vi "Read Mode.vi"(8 "error in (no error)":errorcluster, 11 "Multimeter in":refnum<class "Multimeter.lvclass">) -> (0 "error out":errorcluster, 2 "Mode":T1, 3 "Multimeter out":refnum<class "Multimeter.lvclass">)   [LabVIEW 2019, in "Multimeter.lvlib" / "Multimeter.lvclass"]
uses:
  Library/Multimeter.lvclass
  Custom Controls/Mode.ctl
  Library/Multimeter.lvclass/Multimeter.ctl
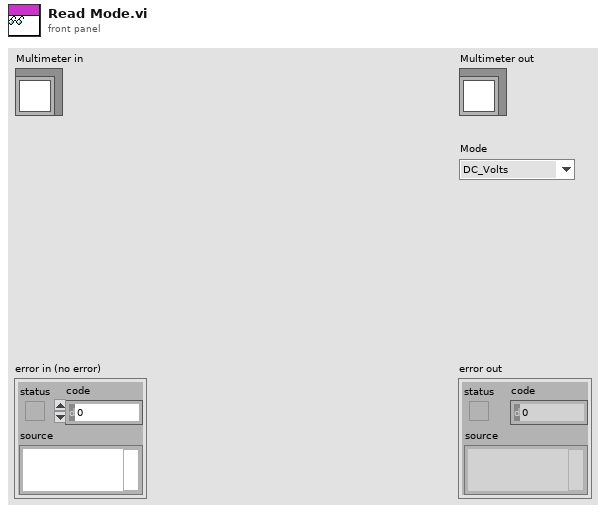
[diagram p1: front panel]
types:
  T1 = typedef "Multimeter.lvlib/Multimeter.lvclass/Mode.ctl" = enum16{"DC_Volts", "AC_Volts", "DC_Current", "AC_Current", "Resistance_2_Wire", "Resistance_4_Wire", "Diode", "Frequency", "Period", "AC_Volts_DC_Coupled", "Capacitance", "Inductance", "Temperature"}
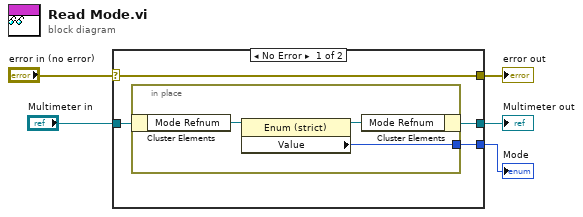
[diagram p0: block diagram]
diagram:
  n1 = case shown="No Error" "error in (no error)" {
    selector: "error in (no error)" -> [w9 w13]
    tunnel: [w9 w13] -> w4
    tunnel: [w7 w14] -> w2
    tunnel: "Multimeter in" -> [w8 w14]
    tunnel: [w6 _] -> w1
    frame No Error {
      n2 = in-place {
        in-place-border: [w10] -> w6
        n3 = in-place-cluster #1(w8) -> ("Mode Refnum"=w12:refnum<vi>)
        n4 = property class="Enum (strict)"(reference=w12) -> (reference out=w11:refnum<vi>, "Value"=w10:T1)  [unwired: 1 in, 1 out]
        n5 = in-place-cluster #1("Mode Refnum"=w11) -> (w7:refnum<class "Multimeter.lvclass">)
      }
    }
    frame Error {
    }
  }
  "error out" <- w4
  "Multimeter out" <- w2
  "Mode" <- w1
